vi "Read Sampling clock.vi"(8 "error in (no error)":errorcluster, 11 "RP Instrument in":refnum<class "RP Instrument.lvclass">) -> (0 "error out":errorcluster, 2 "Sampling clock":T1, 3 "RP Instrument out":refnum<class "RP Instrument.lvclass">)   [LabVIEW 2020, in "RP Instrument.lvclass"]
uses:
  RP Instrument.lvclass
  RP Instrument.lvclass/RP Instrument.ctl
  Controls/Sampling clock.ctl
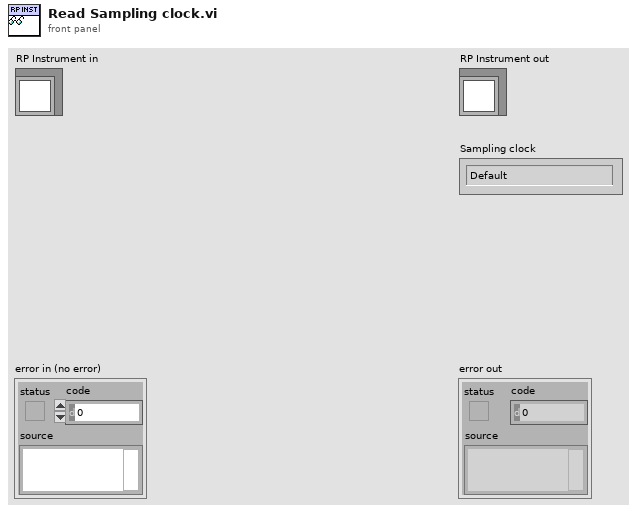
[diagram p1: front panel]
types:
  T1 = typedef "Sampling clock.ctl" = enum16{"Default", "Internal", "Extention connector", "Programmable logic"}
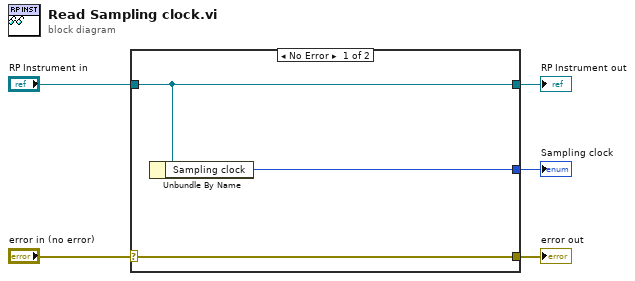
[diagram p0: block diagram]
diagram:
  n1 = case shown="No Error" "error in (no error)" {
    selector: "error in (no error)" -> [w8 w9]
    tunnel: [w8 w9] -> w4
    tunnel: [w7 w10] -> w2
    tunnel: "RP Instrument in" -> [w7 w10]
    tunnel: [w6 _] -> w1
    frame No Error {
      n2 = Unbundle By Name(w7) -> ("Sampling clock"=w6:T1)
    }
    frame Error {
    }
  }
  "error out" <- w4
  "RP Instrument out" <- w2
  "Sampling clock" <- w1
